vi "P´ractica_para_PAI.vi"() -> ()   [LabVIEW 2024]
uses:
  <vilib>/LabVIEW Interface for Arduino/Type Defs/Digital Pin.ctl
  <vilib>/LabVIEW Interface for Arduino/LabVIEW Interface for Arduino.lvlib
panel:
  in  "Detener":bool
  in  "Digital Pin 3":T1
  in  "Digital Pin 2":T1
  in  "Digital Pin":T1
  out "LED 3":bool
  out "LED 2":bool
  out "LED 1":bool
  in  "Interruptor 3":bool
  in  "Interruptor 2":bool
  in  "Interruptor 1":bool
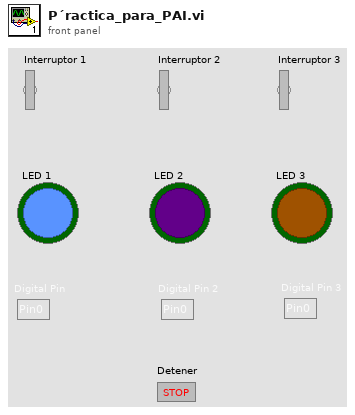
[diagram p1: front panel]
types:
  T1 = typedef "LabVIEW Interface for Arduino.lvlib/Digital Pin.ctl" = enum8{"Pin0", "Pin1", "Pin2", "Pin3", "Pin4", "Pin5", "Pin6", "Pin7", "Pin8", "Pin9", "Pin10", "Pin11", "Pin12", "Pin13"}
  T2 = typedef "LabVIEW Interface for Arduino.lvlib/Arduino Resource.ctl" = cluster{"VISA resource":refnum<visa-resource-name>, "Board Type":T3, "Connection Type":enum8{"USB / Serial"}, "Bytes Per Packet (15)":u8}
  T3 = typedef "LabVIEW Interface for Arduino.lvlib/Board Type.ctl" = enum16{"Uno", "Dimuelanove w/Atmega 328", "Mega 2560"}
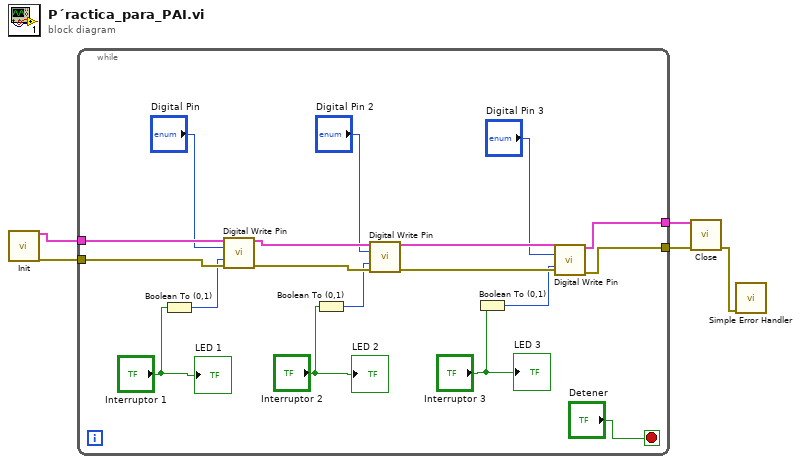
[diagram p0: block diagram]
diagram:
  n1 = call <vilib>:"Init.vi"() -> ("Arduino Resource"=w5:T2, "error out"=w4:errorcluster)  [unwired: 18 in]
  n2 = while {
    tunnel: w5 -> [w23]
    tunnel: w4 -> [w22]
    tunnel: [w17] -> w3
    tunnel: [w16] -> w2
    stop <- "Detener" stop-if-true
    n3 = Boolean To (0,1)(Boolean="Interruptor 1") -> (0, 1=w12:i16)
    n4 = call <vilib>:"Digital Write Pin.vi"("Arduino Resource"=w23, "Digital I/O Pin (0)"="Digital Pin", "Value (0)"=w12, "error in"=w22) -> ("Arduino Resource"=w21:T2, "error out"=w20:errorcluster)  [unwired: 10 in]
    n5 = Boolean To (0,1)(Boolean="Interruptor 2") -> (0, 1=w10:i16)
    n6 = call <vilib>:"Digital Write Pin.vi"("Arduino Resource"=w21, "Digital I/O Pin (0)"="Digital Pin 2", "Value (0)"=w10, "error in"=w20) -> ("Arduino Resource"=w19:T2, "error out"=w18:errorcluster)  [unwired: 10 in]
    n7 = Boolean To (0,1)(Boolean="Interruptor 3") -> (0, 1=w8:i16)
    n8 = call <vilib>:"Digital Write Pin.vi"("Arduino Resource"=w19, "Digital I/O Pin (0)"="Digital Pin 3", "Value (0)"=w8, "error in"=w18) -> ("Arduino Resource"=w17:T2, "error out"=w16:errorcluster)  [unwired: 10 in]
    "LED 2" <- "Interruptor 2"
    "LED 3" <- "Interruptor 3"
    "LED 1" <- "Interruptor 1"
  }
  n9 = call <vilib>:"Close.vi"("Arduino Resource"=w3, "error in"=w2) -> ("error out"=w1:errorcluster)  [unwired: 13 in]
  n10 = call <vilib>:"Simple Error Handler.vi"("error in (no error)"=w1) -> ()  [unwired: 4 in, 5 out]
